vi "speed profile.vi"(10 "Pot position":dbl, 11 "motor speed":dbl) -> (3 "motor output":dbl)   [LabVIEW 2014]
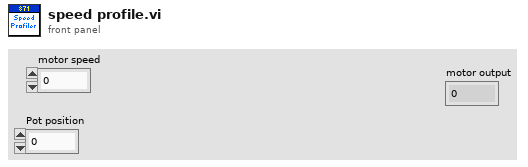
[diagram p1: front panel]
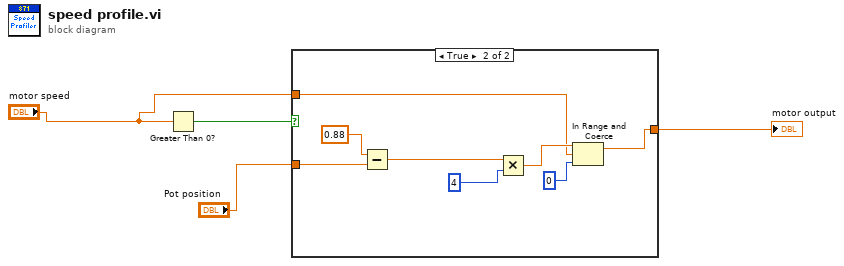
[diagram p0: block diagram]
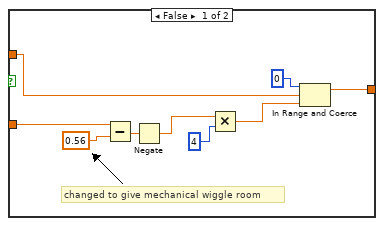
[diagram p2: hidden frame]
diagram:
  n1 = Greater Than 0?(x="motor speed") -> (x > 0?=w3:bool)
  n2 = case shown="True" w3 {
    tunnel: "Pot position" -> [w12 w20]
    tunnel: "motor speed" -> [w7 w16]
    tunnel: [w5 w14] -> w1
    frame False {
      # "changed to give mechanical wiggle room"
      n3 = Subtract(x=w12, y=0.56) -> (x-y=w11:dbl)
      n4 = Negate(x=w11) -> (-x=w9:dbl)
      n5 = Multiply(x=w9, y=4) -> (x*y=w8:dbl)
      n6 = In Range and Coerce(upper limit=0, x=w7, lower limit=w8) -> (coerced(x)=w5:dbl)  [unwired: 1 out]
    }
    frame True {
      n7 = Subtract(x=0.88, y=w20) -> (x-y=w18:dbl)
      n8 = Multiply(x=w18, y=4) -> (x*y=w17:dbl)
      n9 = In Range and Coerce(upper limit=w17, x=w16, lower limit=0) -> (coerced(x)=w14:dbl)  [unwired: 1 out]
    }
  }
  "motor output" <- w1
